vi "FTW-Test-Endpoints.vi"() -> ()   [LabVIEW 2015]
uses:
  source/actor/Ether/FTW-Ether-EndpointType.ctl
  source/actor/Endpoint/FTW-Endpoint.lvclass
  source/actor/Ether/FTW-Ether.lvclass
panel:
  in  "Connection":string(combo)="inproc://*"
  out "Timed out?":bool
  out "Actual Server Address":string
  out "error out":errorcluster
  out "Response Body":string
  out "Response Header":string
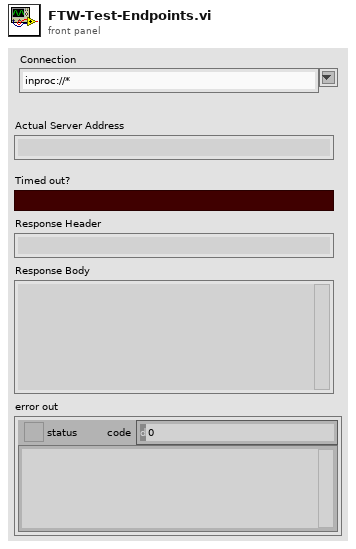
[diagram p1: front panel]
types:
  T1 = typedef "FTW-Ether.lvclass/FTW-Ether-EndpointType.ctl" = enum16{"Server", "Client", "Publisher", "Subscriber"}
  T2 = typedef "FTW-Ether.lvclass/FTW-Ether-MessageTransportScheme.ctl" = enum16{"In process (inproc://)", "TCP (tcp://)"}
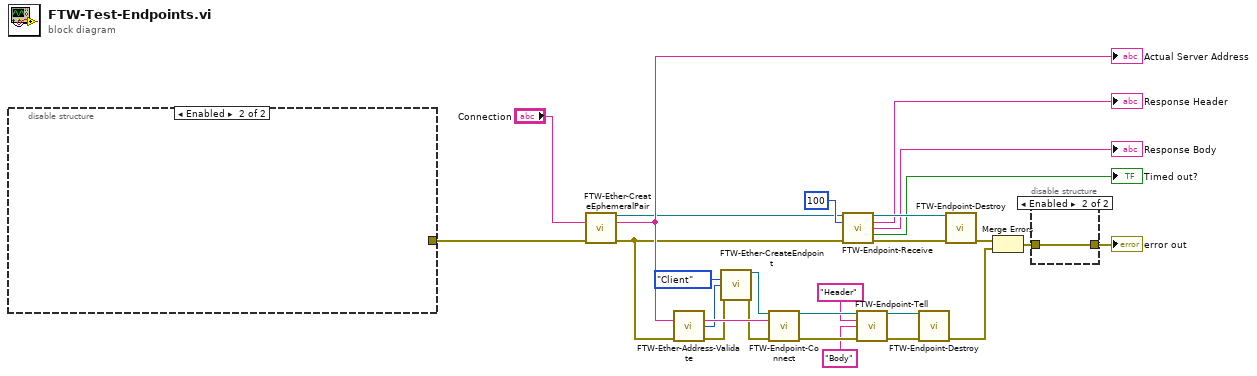
[diagram p0: block diagram]
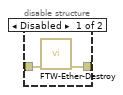
[diagram p2: hidden frame]
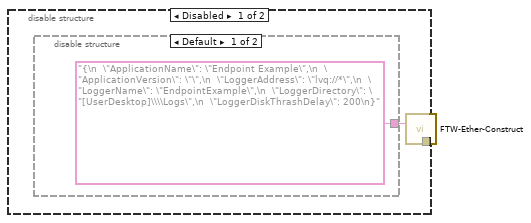
[diagram p3: hidden frame]
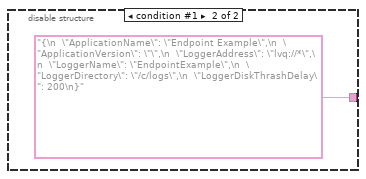
[diagram p4: hidden frame]
diagram:
  n1 = disable-structure shown="Enabled" {
    disable-tunnel: [w28 _] -> w11
    frame Disabled {
      n2 = disable-structure shown="Default" {
        disable-tunnel: ["{\n  \"ApplicationName\": \"Endpoint Example\",\n  \"ApplicationVersion\": \"\",\n  \"LoggerAddress\": \"lvq://*\",\n  \"LoggerName\": \"EndpointExample\",\n  \"LoggerDirectory\": \"[UserDesktop]\\\\Logs\",\n  \"LoggerDiskThrashDelay\": 200\n}" ("FTW Ether Configuration") "{\n  \"ApplicationName\": \"Endpoint Example\",\n  \"ApplicationVersion\": \"\",\n  \"LoggerAddress\": \"lvq://*\",\n  \"LoggerName\": \"EndpointExample\",\n  \"LoggerDirectory\": \"/c/logs\",\n  \"LoggerDiskThrashDelay\": 200\n}" ("FTW Ether Configuration")] -> w29
        frame condition #0 (active) {
        }
        frame condition #1 {
        }
      }
      n3 = call "FTW-Ether-Construct.vi"("FTW Ether Configuration"=w29) -> ("error out"=w28:errorcluster)  [unwired: 14 in]
    }
    frame Enabled {
    }
  }
  n4 = call "FTW-Ether-CreateEphemeralPair.vi"("Requested Ephemeral Address"="Connection", "error in"=w11) -> ("Ephemeral Endpoint"=w9:refnum<class "FTW-Endpoint.lvclass">, "Actual Ephemeral Address"=w10:string, "error out"=w6:errorcluster)  [unwired: 11 in]
  "Actual Server Address" <- w10
  n5 = call "FTW-Ether-Address-Validate.vi"("Address"=w10, "error in"=w6) -> ("Sanitized Address"=w7:string, "Message Transport Scheme"=w2:T2, "error out"=w5:errorcluster)  [unwired: 11 in]
  n6 = call "FTW-Ether-CreateEndpoint.vi"("Endpoint Type"=FTW-Ether-EndpointType."Client", "Message Transport Scheme"=w2, "error in"=w5) -> ("FTW Endpoint"=w3:refnum<class "FTW-Endpoint.lvclass">, "error out"=w4:errorcluster)  [unwired: 11 in]
  n7 = call-dynamic "FTW-Endpoint-Connect.vi"("FTW Endpoint"=w3, "Endpoint Address"=w7, "error in"=w4) -> ("FTW Endpoint out"=w27:refnum<class "FTW-Endpoint.lvclass">, "error out"=w26:errorcluster)  [unwired: 11 in]
  n8 = call-dynamic "FTW-Endpoint-Receive.vi"("FTW Endpoint"=w9, "Timeout"=100, "error in"=w6) -> ("FTW Endpoint out"=w21:refnum<class "FTW-Endpoint.lvclass">, "Message Header"=→"Response Header":string, "Message Body"=→"Response Body":string, "Timed out?"=→"Timed out?":bool, "error out"=w20:errorcluster)  [unwired: 8 in]
  n9 = call-dynamic "FTW-Endpoint-Tell.vi"("FTW Endpoint"=w27, "Message Header"="Header", "Message Body"="Body", "error in"=w26) -> ("FTW Endpoint out"=w23:refnum<class "FTW-Endpoint.lvclass">, "error out"=w22:errorcluster)  [unwired: 9 in, 1 out]
  n10 = call-dynamic "FTW-Endpoint-Destroy.vi"("FTW Endpoint"=w23, "error in"=w22) -> ("error out"=w16:errorcluster)  [unwired: 13 in]
  n11 = call-dynamic "FTW-Endpoint-Destroy.vi"("FTW Endpoint"=w21, "error in"=w20) -> ("error out"=w17:errorcluster)  [unwired: 13 in]
  n12 = Merge Errors(w17, w16) -> (w15:errorcluster)
  n13 = disable-structure shown="Enabled" {
    disable-tunnel: w15 -> [w33 w34]
    disable-tunnel: [w32 w34] -> w14
    frame Disabled {
      n14 = call "FTW-Ether-Destroy.vi"("error in"=w33) -> ("error out"=w32:errorcluster)  [unwired: 14 in]
    }
    frame Enabled {
    }
  }
  "error out" <- w14
